vi "FEA_Model_Build_Cantilever.vi"(11 "FEA_Model in":refnum<class "FEA_Model.lvclass">) -> (3 "FEA_Model out":refnum<class "FEA_Model.lvclass">)   [LabVIEW 2021, in "FEA_Model.lvclass"]
uses:
  FEA_Model.lvclass
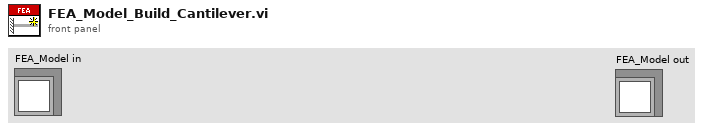
[diagram p1: front panel]
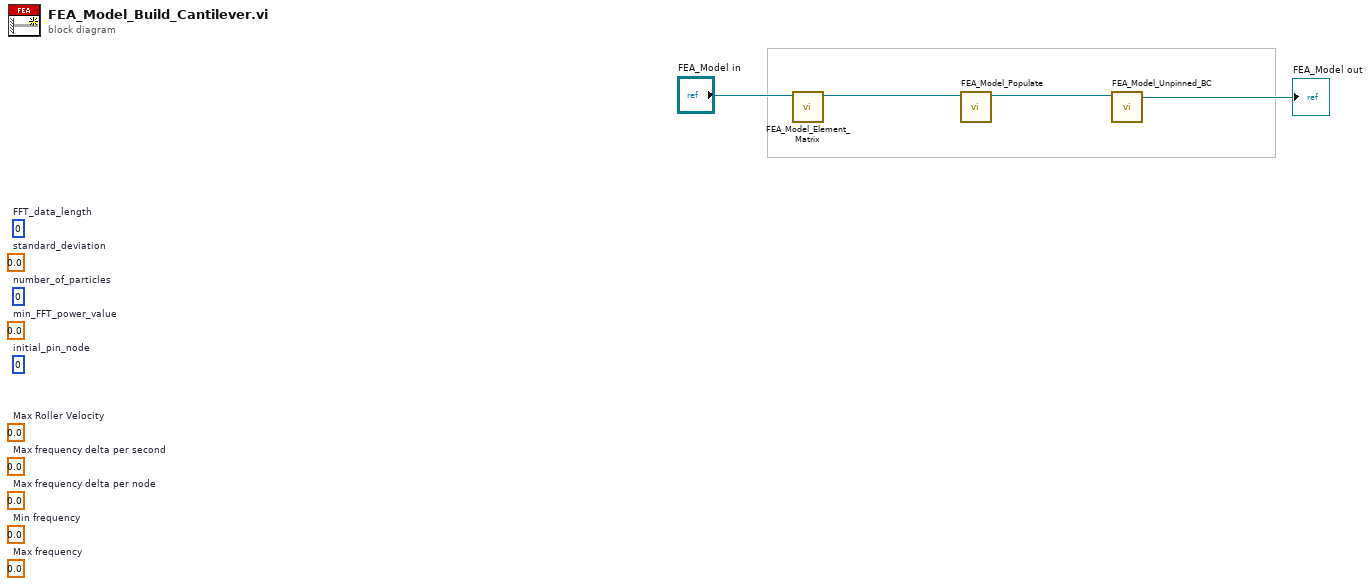
[diagram p0: block diagram]
diagram:
  (unwired) 0  # FFT_data_length
  (unwired) 0.0  # standard_deviation
  (unwired) 0  # number_of_particles
  (unwired) 0.0  # min_FFT_power_value
  (unwired) 0  # initial_pin_node
  (unwired) 0.0  # Max Roller Velocity
  (unwired) 0.0  # Max frequency delta per second
  (unwired) 0.0  # Max frequency delta per node
  (unwired) 0.0  # Min frequency
  (unwired) 0.0  # Max frequency
  n1 = call "FEA_Model_Element_Matrix.vi"("FEA_Model in"="FEA_Model in") -> ("FEA_Model out"=w4:refnum<class "FEA_Model.lvclass">)  [unwired: 10 in]
  n2 = call "FEA_Model_Populate.vi"("FEA_Model in"=w4) -> ("FEA_Model out"=w3:refnum<class "FEA_Model.lvclass">)  [unwired: 10 in]
  n3 = call "FEA_Model_Unpinned_BC.vi"("FEA_Model in"=w3) -> ("FEA_Model out"=→"FEA_Model out":refnum<class "FEA_Model.lvclass">)  [unwired: 10 in]
